vi "sortByTime.vi"(8 "error in (no error)":errorcluster, 10 "data in":T1(array[cluster]), 11 "DeviceData in":refnum<class "DeviceData.lvclass">) -> (0 "error out":errorcluster, 2 "data out":T1(array[cluster]), 3 "DeviceData out":refnum<class "DeviceData.lvclass">)   [LabVIEW 2011, in "DataMappers.lvlib" / "DeviceData.lvclass"]
uses:
  DeviceData.lvclass
  DatabaseHelpers/Database Objects/Channel/Channel.lvclass
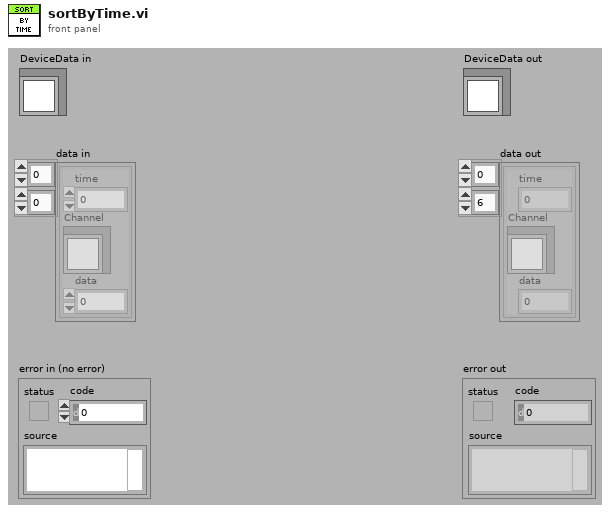
[diagram p1: front panel]
types:
  T1 = cluster{"time":dbl, "Channel":refnum<class "Channel.lvclass">, "data":dbl}[][]
  T2 = cluster{"time":dbl, "Channel":refnum<class "Channel.lvclass">, "data":dbl}[]
  T3 = cluster{"time":dbl, "Channel":refnum<class "Channel.lvclass">, "data":dbl}
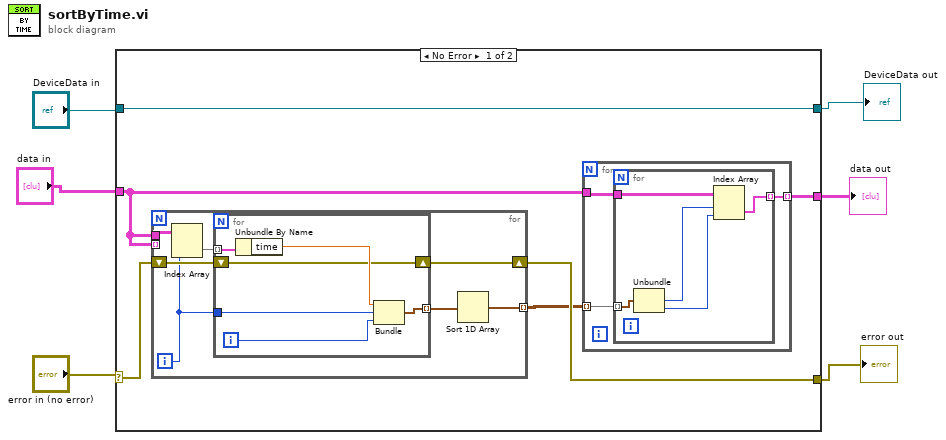
[diagram p0: block diagram]
diagram:
  n1 = case shown="No Error" "error in (no error)" {
    selector: "error in (no error)" -> [w10 w36]
    tunnel: [w9 w36] -> w4
    tunnel: [w12 w35] -> w1
    tunnel: "DeviceData in" -> [w12 w35]
    tunnel: "data in" -> [w7 w34]
    tunnel: [w11 w34] -> w2
    frame No Error {
      n2 = for {
        shift-right: [w26] -> w9
        shift-left: w10 -> [w27]
        tunnel: w7 -> [w25]
        tunnel: [w21] -> w8 mode=indexing
        tunnel: w7 -> [_] mode=indexing
        i -> [w24]
        n3 = Index Array(array=w25, index (row)=w24) -> (element=w23:T2)  [unwired: 1 in]
        n4 = for {
          tunnel: [w33] -> w22 mode=indexing
          tunnel: w24 -> [w31]
          shift-right: [w30] -> w26
          shift-left: w27 -> [w30]
          tunnel: w23 -> [w29] mode=indexing
          i -> [w28]
          n5 = Unbundle By Name(w29) -> ("time"=w32:dbl)
          n6 = Bundle("time"=w32, w31, w28) -> (w33:cluster{"time":dbl, i32, i32})  [unwired: 1 in]
        }
        n7 = Sort 1D Array(array=w22) -> (sorted array=w21:cluster{"time":dbl, i32, i32}[])
      }
      n8 = for {
        tunnel: w8 -> [w13] mode=indexing
        tunnel: w7 -> [w15]
        tunnel: [w14] -> w11 mode=indexing
        n9 = for {
          tunnel: w15 -> [w20]
          tunnel: [w19] -> w14 mode=indexing
          tunnel: w13 -> [w18] mode=indexing
          n10 = Unbundle(w18) -> (w17:i32, w16:i32)  [unwired: 1 out]
          n11 = Index Array(array=w20, index (row)=w17, index (col)=w16) -> (element=w19:T3)
        }
      }
    }
    frame Error {
    }
  }
  "error out" <- w4
  "DeviceData out" <- w1
  "data out" <- w2
